vi "ManualControls_v4.vi"() -> ()   [LabVIEW 2013]
uses:
  <vilib>/Utility/miscctls.llb/LVPointTypeDef.ctl
  <vilib>/DAQmx/write.llb/DAQmx Write (Analog DBL 1Chan 1Samp).vi
  <vilib>/DAQmx/write.llb/DAQmx Write (Digital U32 1Chan 1Samp).vi
  <vilib>/DAQmx/miscellaneous.llb/DAQmx Fill In Error Info.vi
  DeviceVIs/Novatech/Novatech 409A.lvlib
panel:
  in  "Update Hardware":bool
  in  "?":enum32{"Controls", "File IO", "Errors"}(tab)
  in  "Master Output Bits":bool[](array[boolean])=[TRUE, TRUE, TRUE, TRUE, FALSE, FALSE, TRUE, FALSE, FALSE, FALSE, TRUE, FALSE, TRUE, TRUE, TRUE, TRUE, FALSE, FALSE, FALSE, FALSE, FALSE, FALSE, FALSE, FALSE]
  in  "Slave Output Bits":bool[](array[boolean])=[FALSE, FALSE, FALSE, FALSE, FALSE, FALSE, FALSE, FALSE, FALSE, FALSE, FALSE, FALSE, FALSE, FALSE, FALSE, FALSE, FALSE, FALSE, FALSE, FALSE, FALSE, FALSE, FALSE, FALSE]
  in  "Set Master":bool=TRUE
  in  "Set Slave":bool
  in  "AO Values":T1(array[cluster])=[{"DAQmx Global Channel"="AO0_0", "Numeric"=-9.792}, {"DAQmx Global Channel"="AO0_1", "Numeric"=-7.904}, {"DAQmx Global Channel"="AO0_2", "Numeric"=-3.981}, {"DAQmx Global Channel"="AO0_3", "Numeric"=-7.5}, {"DAQmx Global Channel"="AO0_4", "Numeric"=7.0}, {"DAQmx Global Channel"="AO0_5", "Numeric"=1.18}, {"DAQmx Global Channel"="AO0_6", "Numeric"=-8.918}, {"DAQmx Global Channel"="AO0_7", "Numeric"=1.1}, {"DAQmx Global Channel"="AO1_0", "Numeric"=8.0}, {"DAQmx Global Channel"="AO1_1", "Numeric"=0.45}, {"DAQmx Global Channel"="AO1_2", "Numeric"=1.3}, {"DAQmx Global Channel"="AO1_3", "Numeric"=0.0}, {"DAQmx Global Channel"="AO1_4", "Numeric"=0.3}, {"DAQmx Global Channel"="AO1_5", "Numeric"=1.2}, {"DAQmx Global Channel"="AO1_6", "Numeric"=1.6}, {"DAQmx Global Channel"="AO1_7", "Numeric"=0.12}, {"DAQmx Global Channel"="AO2_0", "Numeric"=0.0}, {"DAQmx Global Channel"="AO2_1", "Numeric"=0.0}, {"DAQmx Global Channel"="AO3_0", "Numeric"=0.0}, {"DAQmx Global Channel"="AO3_1", "Numeric"=0.0}, {"DAQmx Global Channel"="AO3_2", "Numeric"=0.0}, {"DAQmx Global Channel"="AO3_3", "Numeric"=0.0}, {"DAQmx Global Channel"="AO3_4", "Numeric"=0.0}, {"DAQmx Global Channel"="AO3_5", "Numeric"=0.0}, {"DAQmx Global Channel"="AO3_6", "Numeric"=0.0}, {"DAQmx Global Channel"="AO3_7", "Numeric"=0.0}] {"Numeric" step=1e-09 format="%_6g"}
  in  "Presets":T2(ring)
  in  "DO Values":T3(array[cluster])=[{"DAQmx Global Channel"="DO0_0", "DO Bits"=[TRUE, TRUE, FALSE, FALSE, FALSE, FALSE, TRUE, TRUE, FALSE, FALSE, FALSE, FALSE, FALSE, FALSE, FALSE, FALSE]}, {"DAQmx Global Channel"="DO1_0", "DO Bits"=[TRUE, FALSE, TRUE, TRUE, FALSE, TRUE, TRUE, TRUE, FALSE, FALSE, FALSE, FALSE, FALSE, FALSE, FALSE, FALSE]}, {"DAQmx Global Channel"="DO2_0", "DO Bits"=[]}, {"DAQmx Global Channel"="DO3_0", "DO Bits"=[]}]
  in  "Novatech settings":T4(array[cluster])
  in  "History":string(combo)
  in  "Save":bool
  in  "Load":bool
  in  "Path":path=path "C:/Experiment/Data Acquisition/Hardware Control/procedures/ManualControl"
  in  "error in":errorcluster
  out "error out":errorcluster
  # "Analog out"
  # "Digital Out"
  # "Ports are setup for 16 bit output, but only 16 are used"
  # "Master PB (PB 0)"
  # "Slave PB (PB 1)"
  # "Novatechs"
  # "0"
  # "8"
  # "12"
  # "4"
  # "16"
  # "20"
  # "0"
  # "8"
  # "12"
  # "4"
  # "16"
  # "20"
  # "Templates"
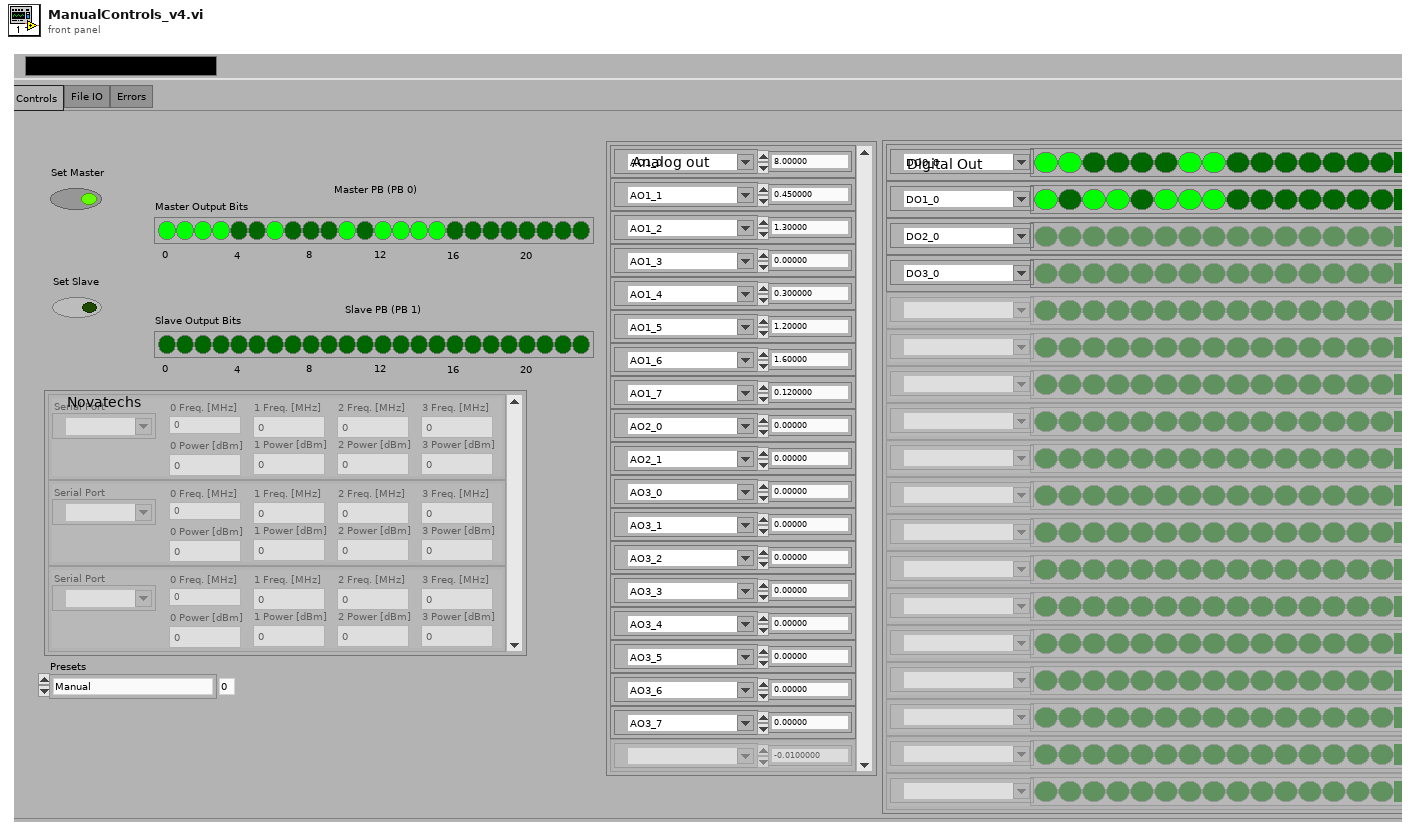
[diagram p1: front panel]
types:
  T1 = cluster{"DAQmx Global Channel":refnum<k21>, "Numeric":dbl}[]
  T2 = enum16{"Manual", "Rb MOT", "Yb MOT", "RbYb Warmup", "RbYb Turn Off", "Sr Warmup"}
  T3 = cluster{"DAQmx Global Channel":refnum<k21>, "DO Bits":bool[]}[]
  T4 = cluster{"0 Freq. [MHz]":dbl, "0 Power [dBm]":dbl, "Serial Port":refnum<visa-resource-name>, "1 Freq. [MHz]":dbl, "1 Power [dBm]":dbl, "2 Freq. [MHz]":dbl, "2 Power [dBm]":dbl, "3 Freq. [MHz]":dbl, "3 Power [dBm]":dbl}[]
  T5 = typedef "Semaphore RefNum" = refnum<k1>
  T6 = enum16{"open", "open or create", "create or replace", "create", "open (read only)"}
  T7 = enum16{"Always On", "Always Off", "Off While Running"}
  T8 = typedef "LVPointTypeDef.ctl" = cluster{"Horizontal":i16, "Vertical":i16}
  T9 = cluster{"Master Output Bits":bool[], "Slave Output Bits":bool[], "AO Values":cluster{"DAQmx Global Channel":refnum<k21>, "Numeric":dbl}[], "DO Values":cluster{"DAQmx Global Channel":refnum<k21>, "DO Bits":bool[]}[], "Novatech settings":cluster{"0 Freq. [MHz]":dbl, "0 Power [dBm]":dbl, "Serial Port":refnum<visa-resource-name>, "1 Freq. [MHz]":dbl, "1 Power [dBm]":dbl, "2 Freq. [MHz]":dbl, "2 Power [dBm]":dbl, "3 Freq. [MHz]":dbl, "3 Power [dBm]":dbl}[]}
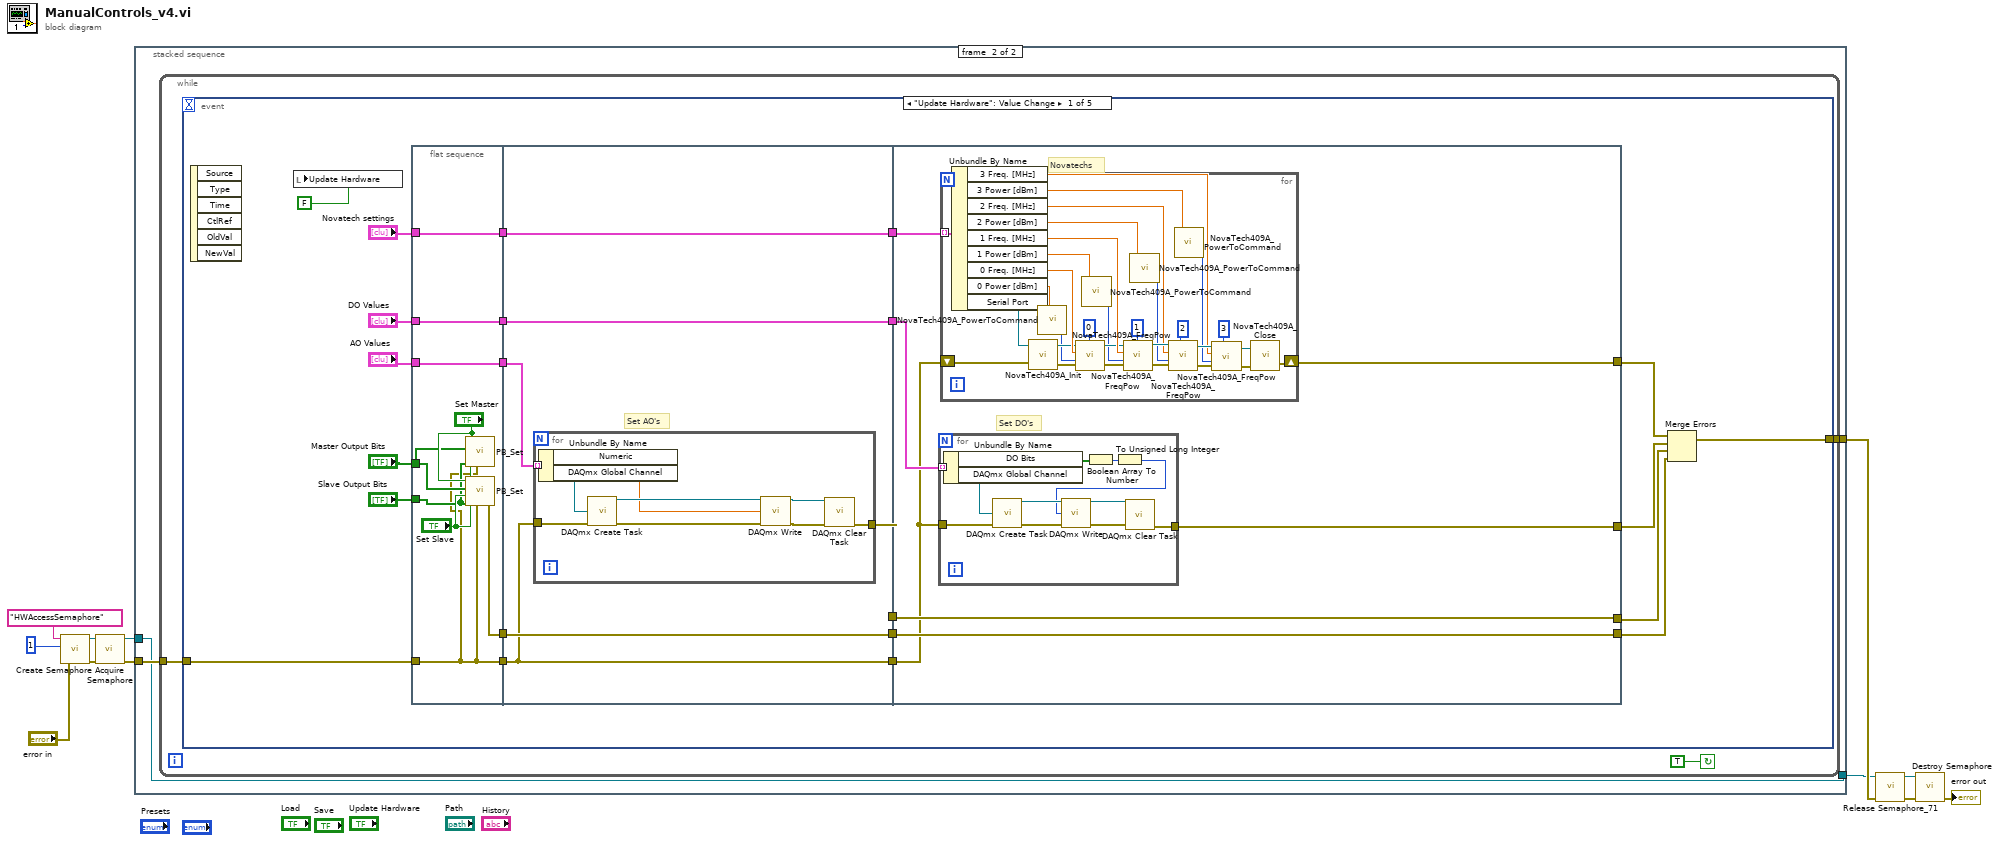
[diagram p0: block diagram]
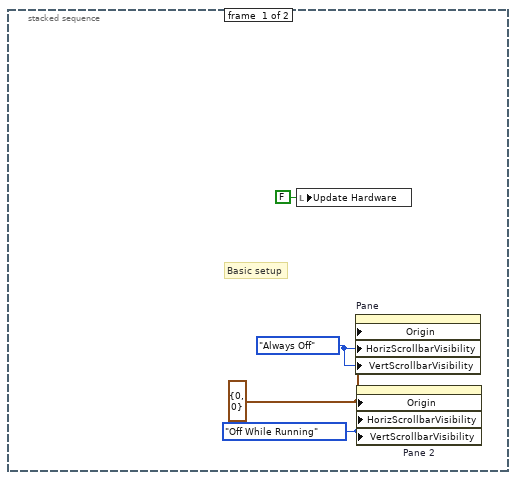
[diagram p2: hidden frame]
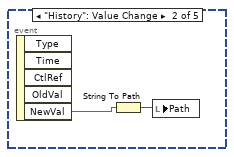
[diagram p3: hidden frame]
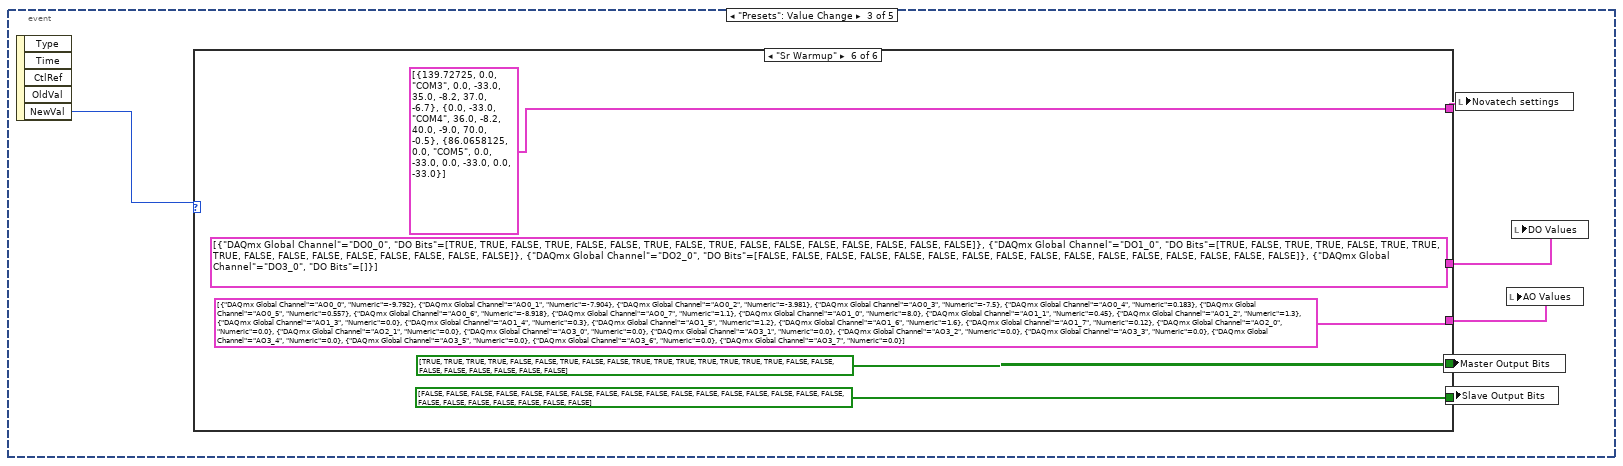
[diagram p4: hidden frame]
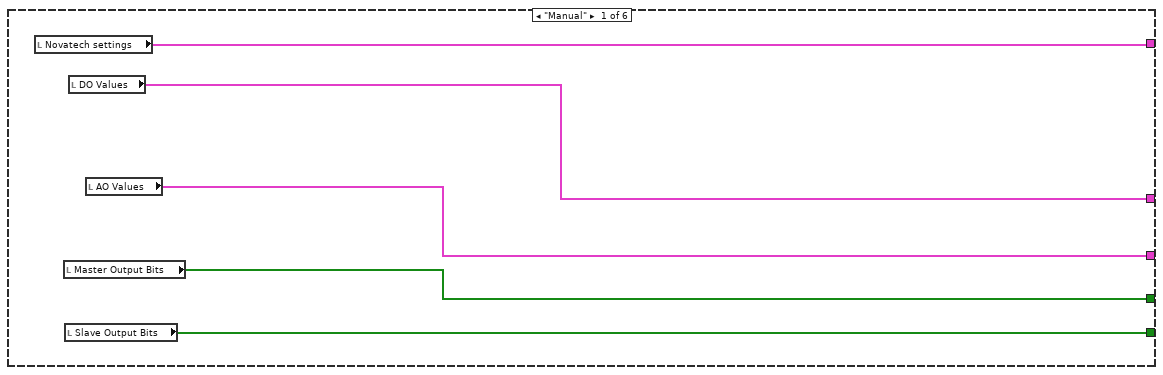
[diagram p5: hidden frame]
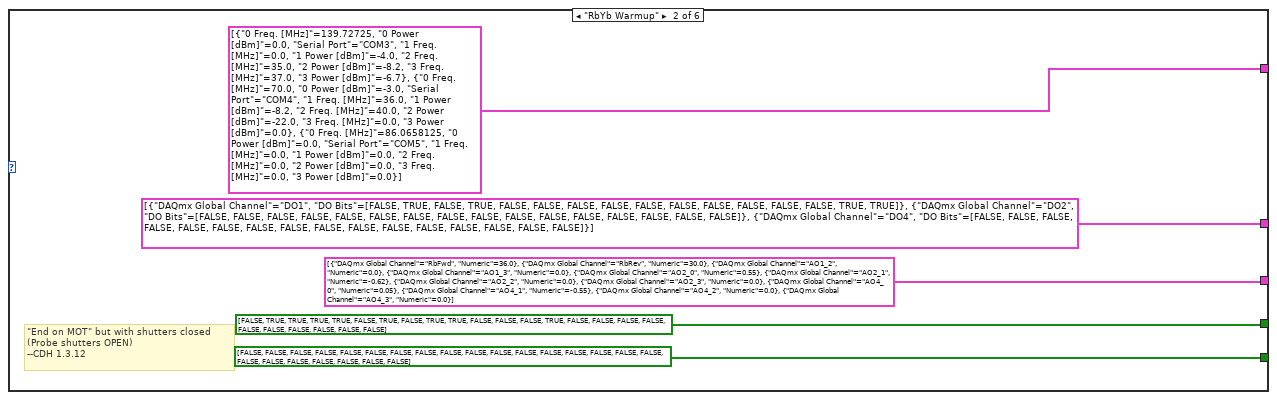
[diagram p6: hidden frame]
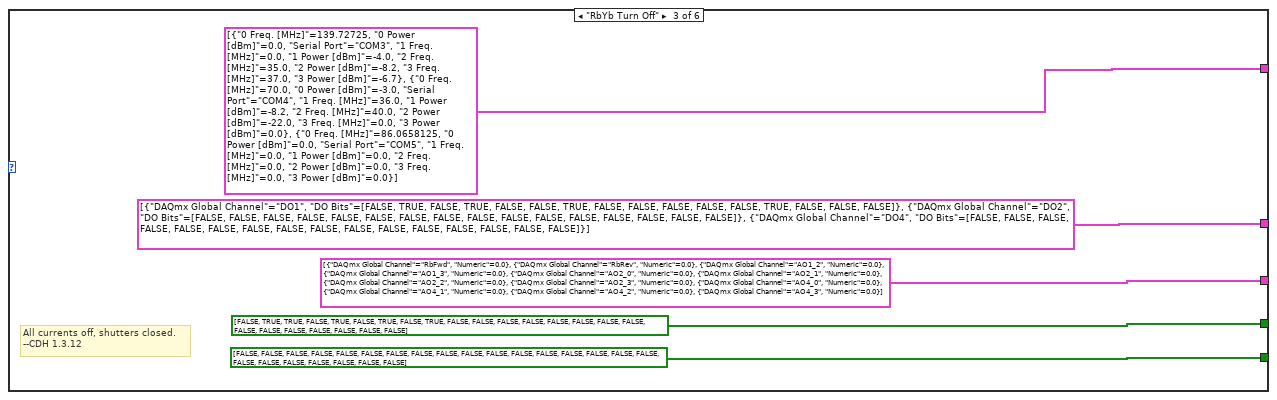
[diagram p7: hidden frame]
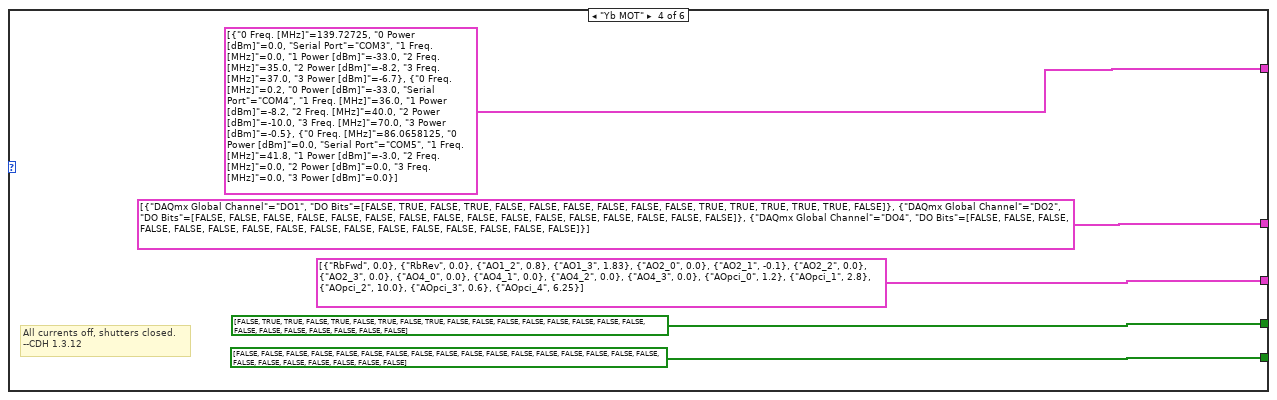
[diagram p8: hidden frame]
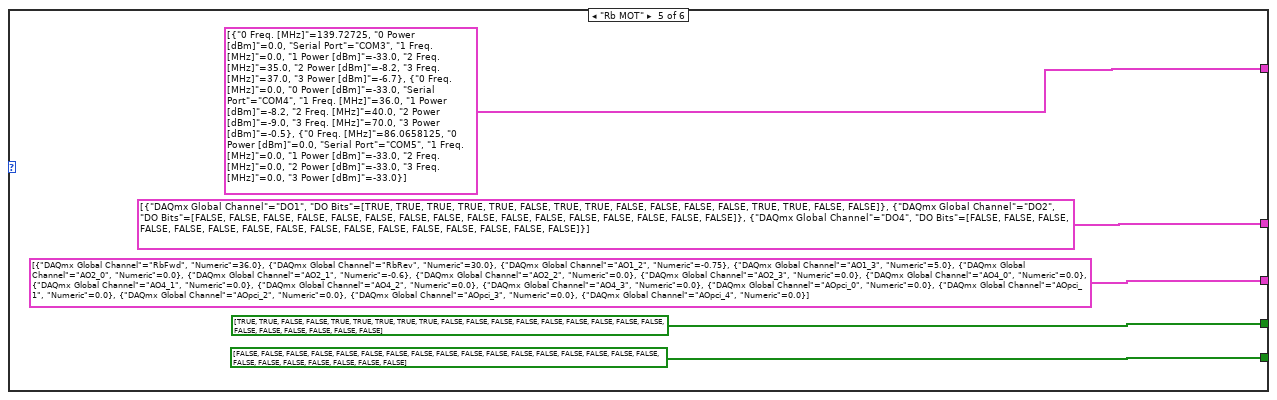
[diagram p9: hidden frame]
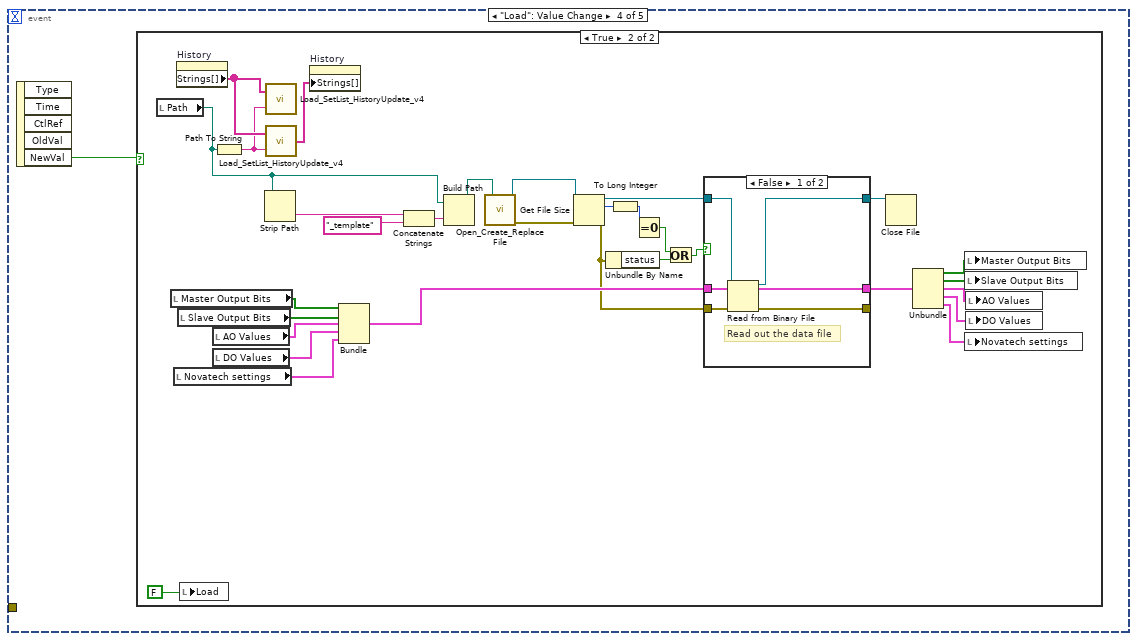
[diagram p10: hidden frame]
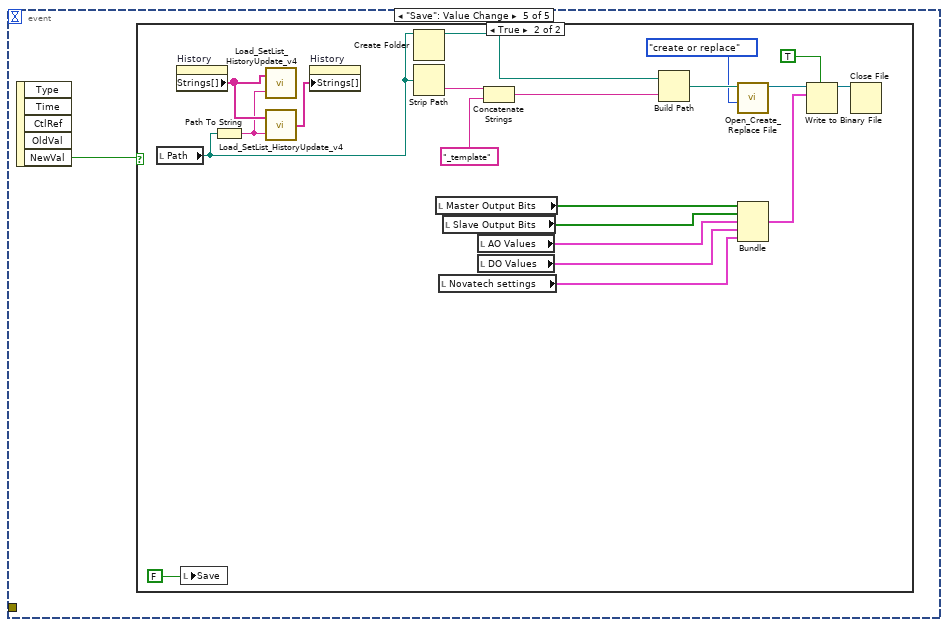
[diagram p13: hidden frame]
diagram:
  n1 = call <vilib>:"Create Semaphore.vi"("error in (no error)"="error in", "size (1)"=1, "name (unnamed)"="HWAccessSemaphore") -> ("error out"=w6:errorcluster, "semaphore"=w7:T5)  [unwired: 3 out]
  n2 = call <vilib>:"Acquire Semaphore.vi"("error in (no error)"=w6, "semaphore"=w7) -> ("error out"=w3:errorcluster, "semaphore out"=w2:T5)  [unwired: 1 in, 3 out]
  n3 = stacked-sequence {
    tunnel: [_ w19] -> w9
    tunnel: w3 -> [_ w18]
    tunnel: w2 -> [_ w17]
    tunnel: [_ w17] -> w1
    frame #0 {
      w16 = T7."Always Off" ("Horizontal Scrollbar Visibility")
      w15 = T8 {"Horizontal"=0, "Vertical"=0} ("Origin")
      w14 = T7."Off While Running" ("Horizontal Scrollbar Visibility")
      # "Basic setup"
      n4 = local write "Update Hardware"(FALSE ("Update Hardware")) -> ()
      n5 = property on="Pane" class="Pane"("Origin"=w15, "HorizScrollbarVisibility"=w16, "VertScrollbarVisibility"=w16) -> ()  [unwired: 2 in, 2 out]
      n6 = property on="Pane 2" class="Pane"("Origin"=w15, "HorizScrollbarVisibility"=w14, "VertScrollbarVisibility"=w14) -> ()  [unwired: 2 in, 2 out]
    }
    frame #1 {
      n7 = while {
        tunnel: [w22] -> w19
        tunnel: w18 -> [w21]
        stop <- TRUE continue-if-true
        n8 = event shown="[0] \"Update Hardware\": Value Change" {
          selector: _ -> [_ _ _ _ _]
          dyn-events: _ -> [_ _ _ _ _]
          timeout: _ -> [_ _ _ _ _]
          tunnel: [w44 _ _ _ _] -> w22
          tunnel: w21 -> [w43 _ _ _ _]
          event "Update Hardware": Value Change {
            n9 = event-data() -> ()  [unwired: 1 in, 6 out]
            n10 = local write "Update Hardware"(FALSE) -> ()
            n11 = flat-sequence {
              tunnel: [w45] -> w42
              tunnel: [w51] -> w41
              tunnel: "AO Values" -> [w51]
              tunnel: "Master Output Bits" -> [w50]
              tunnel: "Slave Output Bits" -> [w49]
              tunnel: "DO Values" -> [w47]
              tunnel: "Novatech settings" -> [w48]
              tunnel: [w47] -> w40
              tunnel: [w48] -> w39
              tunnel: w43 -> [w46]
              tunnel: [w46] -> w38
              tunnel: w42 -> [w55]
              tunnel: w41 -> [w58]
              tunnel: [w59] -> w37
              tunnel: w40 -> [w57]
              tunnel: [w57] -> w36
              tunnel: [w56] -> w35
              tunnel: w39 -> [w56]
              tunnel: [w54] -> w34
              tunnel: w38 -> [w54]
              tunnel: [w55] -> w33
              tunnel: [w75] -> w31
              tunnel: w37 -> [w70]
              tunnel: w36 -> [w74]
              tunnel: [w73] -> w32
              tunnel: w35 -> [w72]
              tunnel: w34 -> [w69]
              tunnel: [w71] -> w24
              tunnel: w33 -> [w71]
              tunnel: [w70] -> w25
              frame #0 {
                # "Set PulseBlaster"
                n12 = call "PB_Set.vi"("Set Master"="Set Master", "Master Output Bits"=w50, "Set Slave"="Set Slave", "Slave Output Bits"=w49, "error in"=w46) -> ()  [unwired: 3 out]
                n13 = call "PB_Set.vi"("Set Master"="Set Master", "Master Output Bits"=w50, "Set Slave"="Set Slave", "Slave Output Bits"=w49, "error in"=w46) -> ("error out"=w45:errorcluster)  [unwired: 2 out]
              }
              frame #1 {
                # "Set AO's"
                n14 = for {
                  tunnel: [w66] -> w59
                  tunnel: w54 -> [w65]
                  tunnel: w58 -> [w62] mode=indexing
                  n15 = Unbundle By Name(w62) -> ("Numeric"=w61:dbl, "DAQmx Global Channel"=w60:refnum<k21>)
                  n16 = call <vilib>:"DAQmx Create Task.vi"("global virtual channels"=w60, "error in"=w65) -> ("task out"=w63:refnum<k21>, "error out"=w64:errorcluster)  [unwired: 3 in, 9 out]
                  n17 = call-poly <vilib>:"DAQmx Write.vi"("task/channels in"=w63, "data"=w61, "error in"=w64) -> ("task out"=w68:refnum<k21>, "error out"=w67:errorcluster)  [unwired: 1 in, 10 out]
                  n18 = call <vilib>:"DAQmx Clear Task.vi"("task in"=w68, "error in"=w67) -> ("error out"=w66:errorcluster)  [unwired: 13 out]
                }
              }
              frame #2 {
                # "Novatechs"
                # "Set DO's"
                n19 = for {
                  tunnel: [w114] -> w75
                  tunnel: w69 -> [w113]
                  tunnel: w74 -> [w110] mode=indexing
                  n20 = Unbundle By Name(w110) -> ("DO Bits"=w107:bool[], "DAQmx Global Channel"=w109:refnum<k21>)
                  n21 = call <vilib>:"DAQmx Create Task.vi"("global virtual channels"=w109, "error in"=w113) -> ("task out"=w111:refnum<k21>, "error out"=w112:errorcluster)  [unwired: 3 in, 9 out]
                  n22 = Boolean Array To Number(Boolean array=w107) -> (number=w108:u32)
                  n23 = To Unsigned Long Integer(number=w108) -> (unsigned 32bit integer=w106:u32)
                  n24 = call-poly <vilib>:"DAQmx Write.vi"("task/channels in"=w111, "data"=w106, "error in"=w112) -> ("task out"=w116:refnum<k21>, "error out"=w115:errorcluster)  [unwired: 1 in, 10 out]
                  n25 = call <vilib>:"DAQmx Clear Task.vi"("task in"=w116, "error in"=w115) -> ("error out"=w114:errorcluster)  [unwired: 13 out]
                }
                n26 = for {
                  tunnel: w72 -> [w105] mode=indexing
                  shift-right: [w91] -> w73
                  shift-left: w69 -> [w103]
                  n27 = Unbundle By Name(w105) -> ("3 Freq. [MHz]"=w84:dbl, "3 Power [dBm]"=w83:dbl, "2 Freq. [MHz]"=w85:dbl, "2 Power [dBm]"=w80:dbl, "1 Freq. [MHz]"=w98:dbl, "1 Power [dBm]"=w78:dbl, "0 Freq. [MHz]"=w100:dbl, "0 Power [dBm]"=w76:dbl, "Serial Port"=w104:refnum<visa-resource-name>)
                  n28 = call "NovaTech409A_Init.vi"("error in (no error)"=w103, "VISA resource name"=w104) -> ("error out"=w102:errorcluster, "VISA resource name out"=w99:refnum<visa-resource-name>)  [unwired: 1 in]
                  n29 = call "NovaTech409A_PowerToCommand.vi"("Novatech Power [dBm]"=w76) -> ("Novatech Command"=w77:u16)
                  n30 = call "NovaTech409A_FreqPow.vi"("VISA resource name"=w99, "Freq"=w100, "Power"=w77, "error in (no error)"=w102, "Channel (0-3)"=u8 0) -> ("VISA resource name out"=w97:refnum<visa-resource-name>, "error out"=w101:errorcluster)
                  n31 = call "NovaTech409A_PowerToCommand.vi"("Novatech Power [dBm]"=w78) -> ("Novatech Command"=w79:u16)
                  n32 = call "NovaTech409A_FreqPow.vi"("VISA resource name"=w97, "Freq"=w98, "Power"=w79, "error in (no error)"=w101, "Channel (0-3)"=u8 1) -> ("VISA resource name out"=w90:refnum<visa-resource-name>, "error out"=w94:errorcluster)
                  n33 = call "NovaTech409A_PowerToCommand.vi"("Novatech Power [dBm]"=w80) -> ("Novatech Command"=w81:u16)
                  n34 = call "NovaTech409A_FreqPow.vi"("VISA resource name"=w90, "Freq"=w85, "Power"=w81, "error in (no error)"=w94, "Channel (0-3)"=u8 2) -> ("VISA resource name out"=w89:refnum<visa-resource-name>, "error out"=w93:errorcluster)
                  n35 = call "NovaTech409A_PowerToCommand.vi"("Novatech Power [dBm]"=w83) -> ("Novatech Command"=w82:u16)
                  n36 = call "NovaTech409A_FreqPow.vi"("VISA resource name"=w89, "Freq"=w84, "Power"=w82, "error in (no error)"=w93, "Channel (0-3)"=u8 3) -> ("VISA resource name out"=w88:refnum<visa-resource-name>, "error out"=w92:errorcluster)
                  n37 = call "NovaTech409A_Close.vi"("error in (no error)"=w92, "VISA resource name"=w88) -> ("error out"=w91:errorcluster)  [unwired: 1 out]
                }
              }
            }
            n38 = Merge Errors(w32, w31, w25, w24) -> (w44:errorcluster)
          }
          event "History": Value Change {
            n39 = event-data() -> ("NewVal"=w118:string)  [unwired: 1 in, 4 out]
            n40 = String To Path(string=w118) -> (path=w117:path)
            n41 = local write "Path"(w117) -> ()
          }
          event "Presets": Value Change {
            n42 = event-data() -> ("NewVal"=w119:T2)  [unwired: 1 in, 4 out]
            n43 = case shown="\"Sr Warmup\"" w119 {
              tunnel: [w127 T1 [{"DAQmx Global Channel"="RbFwd", "Numeric"=36.0}, {"DAQmx Global Channel"="RbRev", "Numeric"=30.0}, {"DAQmx Global Channel"="AO1_2", "Numeric"=0.0}, {"DAQmx Global Channel"="AO1_3", "Numeric"=0.0}, {"DAQmx Global Channel"="AO2_0", "Numeric"=0.55}, {"DAQmx Global Channel"="AO2_1", "Numeric"=-0.62}, {"DAQmx Global Channel"="AO2_2", "Numeric"=0.0}, {"DAQmx Global Channel"="AO2_3", "Numeric"=0.0}, {"DAQmx Global Channel"="AO4_0", "Numeric"=0.05}, {"DAQmx Global Channel"="AO4_1", "Numeric"=-0.55}, {"DAQmx Global Channel"="AO4_2", "Numeric"=0.0}, {"DAQmx Global Channel"="AO4_3", "Numeric"=0.0}] ("AO Values") T1 [{"DAQmx Global Channel"="RbFwd", "Numeric"=0.0}, {"DAQmx Global Channel"="RbRev", "Numeric"=0.0}, {"DAQmx Global Channel"="AO1_2", "Numeric"=0.0}, {"DAQmx Global Channel"="AO1_3", "Numeric"=0.0}, {"DAQmx Global Channel"="AO2_0", "Numeric"=0.0}, {"DAQmx Global Channel"="AO2_1", "Numeric"=0.0}, {"DAQmx Global Channel"="AO2_2", "Numeric"=0.0}, {"DAQmx Global Channel"="AO2_3", "Numeric"=0.0}, {"DAQmx Global Channel"="AO4_0", "Numeric"=0.0}, {"DAQmx Global Channel"="AO4_1", "Numeric"=0.0}, {"DAQmx Global Channel"="AO4_2", "Numeric"=0.0}, {"DAQmx Global Channel"="AO4_3", "Numeric"=0.0}] ("AO Values") T1 [{"DAQmx Global Channel"="RbFwd", "Numeric"=0.0}, {"DAQmx Global Channel"="RbRev", "Numeric"=0.0}, {"DAQmx Global Channel"="AO1_2", "Numeric"=0.8}, {"DAQmx Global Channel"="AO1_3", "Numeric"=1.83}, {"DAQmx Global Channel"="AO2_0", "Numeric"=0.0}, {"DAQmx Global Channel"="AO2_1", "Numeric"=-0.1}, {"DAQmx Global Channel"="AO2_2", "Numeric"=0.0}, {"DAQmx Global Channel"="AO2_3", "Numeric"=0.0}, {"DAQmx Global Channel"="AO4_0", "Numeric"=0.0}, {"DAQmx Global Channel"="AO4_1", "Numeric"=0.0}, {"DAQmx Global Channel"="AO4_2", "Numeric"=0.0}, {"DAQmx Global Channel"="AO4_3", "Numeric"=0.0}, {"DAQmx Global Channel"="AOpci_0", "Numeric"=1.2}, {"DAQmx Global Channel"="AOpci_1", "Numeric"=2.8}, {"DAQmx Global Channel"="AOpci_2", "Numeric"=10.0}, {"DAQmx Global Channel"="AOpci_3", "Numeric"=0.6}, {"DAQmx Global Channel"="AOpci_4", "Numeric"=6.25}] ("AO Values") T1 [{"DAQmx Global Channel"="RbFwd", "Numeric"=36.0}, {"DAQmx Global Channel"="RbRev", "Numeric"=30.0}, {"DAQmx Global Channel"="AO1_2", "Numeric"=-0.75}, {"DAQmx Global Channel"="AO1_3", "Numeric"=5.0}, {"DAQmx Global Channel"="AO2_0", "Numeric"=0.0}, {"DAQmx Global Channel"="AO2_1", "Numeric"=-0.6}, {"DAQmx Global Channel"="AO2_2", "Numeric"=0.0}, {"DAQmx Global Channel"="AO2_3", "Numeric"=0.0}, {"DAQmx Global Channel"="AO4_0", "Numeric"=0.0}, {"DAQmx Global Channel"="AO4_1", "Numeric"=0.0}, {"DAQmx Global Channel"="AO4_2", "Numeric"=0.0}, {"DAQmx Global Channel"="AO4_3", "Numeric"=0.0}, {"DAQmx Global Channel"="AOpci_0", "Numeric"=0.0}, {"DAQmx Global Channel"="AOpci_1", "Numeric"=0.0}, {"DAQmx Global Channel"="AOpci_2", "Numeric"=0.0}, {"DAQmx Global Channel"="AOpci_3", "Numeric"=0.0}, {"DAQmx Global Channel"="AOpci_4", "Numeric"=0.0}] ("AO Values") T1 [{"DAQmx Global Channel"="AO0_0", "Numeric"=-9.792}, {"DAQmx Global Channel"="AO0_1", "Numeric"=-7.904}, {"DAQmx Global Channel"="AO0_2", "Numeric"=-3.981}, {"DAQmx Global Channel"="AO0_3", "Numeric"=-7.5}, {"DAQmx Global Channel"="AO0_4", "Numeric"=0.183}, {"DAQmx Global Channel"="AO0_5", "Numeric"=0.557}, {"DAQmx Global Channel"="AO0_6", "Numeric"=-8.918}, {"DAQmx Global Channel"="AO0_7", "Numeric"=1.1}, {"DAQmx Global Channel"="AO1_0", "Numeric"=8.0}, {"DAQmx Global Channel"="AO1_1", "Numeric"=0.45}, {"DAQmx Global Channel"="AO1_2", "Numeric"=1.3}, {"DAQmx Global Channel"="AO1_3", "Numeric"=0.0}, {"DAQmx Global Channel"="AO1_4", "Numeric"=0.3}, {"DAQmx Global Channel"="AO1_5", "Numeric"=1.2}, {"DAQmx Global Channel"="AO1_6", "Numeric"=1.6}, {"DAQmx Global Channel"="AO1_7", "Numeric"=0.12}, {"DAQmx Global Channel"="AO2_0", "Numeric"=0.0}, {"DAQmx Global Channel"="AO2_1", "Numeric"=0.0}, {"DAQmx Global Channel"="AO3_0", "Numeric"=0.0}, {"DAQmx Global Channel"="AO3_1", "Numeric"=0.0}, {"DAQmx Global Channel"="AO3_2", "Numeric"=0.0}, {"DAQmx Global Channel"="AO3_3", "Numeric"=0.0}, {"DAQmx Global Channel"="AO3_4", "Numeric"=0.0}, {"DAQmx Global Channel"="AO3_5", "Numeric"=0.0}, {"DAQmx Global Channel"="AO3_6", "Numeric"=0.0}, {"DAQmx Global Channel"="AO3_7", "Numeric"=0.0}] ("AO Values")] -> w122
              tunnel: [w126 bool[] [FALSE, TRUE, TRUE, TRUE, TRUE, FALSE, TRUE, FALSE, TRUE, TRUE, FALSE, FALSE, FALSE, TRUE, FALSE, FALSE, FALSE, FALSE, FALSE, FALSE, FALSE, FALSE, FALSE, FALSE] ("Master Output Bits") bool[] [FALSE, TRUE, TRUE, FALSE, TRUE, FALSE, TRUE, FALSE, TRUE, FALSE, FALSE, FALSE, FALSE, FALSE, FALSE, FALSE, FALSE, FALSE, FALSE, FALSE, FALSE, FALSE, FALSE, FALSE] ("Master Output Bits") bool[] [FALSE, TRUE, TRUE, FALSE, TRUE, FALSE, TRUE, FALSE, TRUE, FALSE, FALSE, FALSE, FALSE, FALSE, FALSE, FALSE, FALSE, FALSE, FALSE, FALSE, FALSE, FALSE, FALSE, FALSE] ("Master Output Bits") bool[] [TRUE, TRUE, FALSE, FALSE, TRUE, TRUE, TRUE, TRUE, TRUE, FALSE, FALSE, FALSE, FALSE, FALSE, FALSE, FALSE, FALSE, FALSE, FALSE, FALSE, FALSE, FALSE, FALSE, FALSE] ("Master Output Bits") bool[] [TRUE, TRUE, TRUE, TRUE, FALSE, FALSE, TRUE, FALSE, FALSE, TRUE, TRUE, TRUE, TRUE, TRUE, TRUE, TRUE, FALSE, FALSE, FALSE, FALSE, FALSE, FALSE, FALSE, FALSE] ("Master Output Bits")] -> w120
              tunnel: [w125 bool[] [FALSE, FALSE, FALSE, FALSE, FALSE, FALSE, FALSE, FALSE, FALSE, FALSE, FALSE, FALSE, FALSE, FALSE, FALSE, FALSE, FALSE, FALSE, FALSE, FALSE, FALSE, FALSE, FALSE, FALSE] ("Slave Output Bits") bool[] [FALSE, FALSE, FALSE, FALSE, FALSE, FALSE, FALSE, FALSE, FALSE, FALSE, FALSE, FALSE, FALSE, FALSE, FALSE, FALSE, FALSE, FALSE, FALSE, FALSE, FALSE, FALSE, FALSE, FALSE] ("Slave Output Bits") bool[] [FALSE, FALSE, FALSE, FALSE, FALSE, FALSE, FALSE, FALSE, FALSE, FALSE, FALSE, FALSE, FALSE, FALSE, FALSE, FALSE, FALSE, FALSE, FALSE, FALSE, FALSE, FALSE, FALSE, FALSE] ("Slave Output Bits") bool[] [FALSE, FALSE, FALSE, FALSE, FALSE, FALSE, FALSE, FALSE, FALSE, FALSE, FALSE, FALSE, FALSE, FALSE, FALSE, FALSE, FALSE, FALSE, FALSE, FALSE, FALSE, FALSE, FALSE, FALSE] ("Slave Output Bits") bool[] [FALSE, FALSE, FALSE, FALSE, FALSE, FALSE, FALSE, FALSE, FALSE, FALSE, FALSE, FALSE, FALSE, FALSE, FALSE, FALSE, FALSE, FALSE, FALSE, FALSE, FALSE, FALSE, FALSE, FALSE] ("Slave Output Bits")] -> w121
              tunnel: [w128 T3 [{"DAQmx Global Channel"="DO1", "DO Bits"=[FALSE, TRUE, FALSE, TRUE, FALSE, FALSE, FALSE, FALSE, FALSE, FALSE, FALSE, FALSE, FALSE, FALSE, TRUE, TRUE]}, {"DAQmx Global Channel"="DO2", "DO Bits"=[FALSE, FALSE, FALSE, FALSE, FALSE, FALSE, FALSE, FALSE, FALSE, FALSE, FALSE, FALSE, FALSE, FALSE, FALSE, FALSE]}, {"DAQmx Global Channel"="DO4", "DO Bits"=[FALSE, FALSE, FALSE, FALSE, FALSE, FALSE, FALSE, FALSE, FALSE, FALSE, FALSE, FALSE, FALSE, FALSE, FALSE, FALSE]}] ("DO Values") T3 [{"DAQmx Global Channel"="DO1", "DO Bits"=[FALSE, TRUE, FALSE, TRUE, FALSE, FALSE, TRUE, FALSE, FALSE, FALSE, FALSE, FALSE, TRUE, FALSE, FALSE, FALSE]}, {"DAQmx Global Channel"="DO2", "DO Bits"=[FALSE, FALSE, FALSE, FALSE, FALSE, FALSE, FALSE, FALSE, FALSE, FALSE, FALSE, FALSE, FALSE, FALSE, FALSE, FALSE]}, {"DAQmx Global Channel"="DO4", "DO Bits"=[FALSE, FALSE, FALSE, FALSE, FALSE, FALSE, FALSE, FALSE, FALSE, FALSE, FALSE, FALSE, FALSE, FALSE, FALSE, FALSE]}] ("DO Values") T3 [{"DAQmx Global Channel"="DO1", "DO Bits"=[FALSE, TRUE, FALSE, TRUE, FALSE, FALSE, FALSE, FALSE, FALSE, FALSE, TRUE, TRUE, TRUE, TRUE, TRUE, FALSE]}, {"DAQmx Global Channel"="DO2", "DO Bits"=[FALSE, FALSE, FALSE, FALSE, FALSE, FALSE, FALSE, FALSE, FALSE, FALSE, FALSE, FALSE, FALSE, FALSE, FALSE, FALSE]}, {"DAQmx Global Channel"="DO4", "DO Bits"=[FALSE, FALSE, FALSE, FALSE, FALSE, FALSE, FALSE, FALSE, FALSE, FALSE, FALSE, FALSE, FALSE, FALSE, FALSE, FALSE]}] ("DO Values") T3 [{"DAQmx Global Channel"="DO1", "DO Bits"=[TRUE, TRUE, TRUE, TRUE, TRUE, FALSE, TRUE, TRUE, FALSE, FALSE, FALSE, FALSE, TRUE, TRUE, FALSE, FALSE]}, {"DAQmx Global Channel"="DO2", "DO Bits"=[FALSE, FALSE, FALSE, FALSE, FALSE, FALSE, FALSE, FALSE, FALSE, FALSE, FALSE, FALSE, FALSE, FALSE, FALSE, FALSE]}, {"DAQmx Global Channel"="DO4", "DO Bits"=[FALSE, FALSE, FALSE, FALSE, FALSE, FALSE, FALSE, FALSE, FALSE, FALSE, FALSE, FALSE, FALSE, FALSE, FALSE, FALSE]}] ("DO Values") T3 [{"DAQmx Global Channel"="DO0_0", "DO Bits"=[TRUE, TRUE, FALSE, TRUE, FALSE, FALSE, TRUE, FALSE, TRUE, FALSE, FALSE, FALSE, FALSE, FALSE, FALSE, FALSE]}, {"DAQmx Global Channel"="DO1_0", "DO Bits"=[TRUE, FALSE, TRUE, TRUE, FALSE, TRUE, TRUE, TRUE, FALSE, FALSE, FALSE, FALSE, FALSE, FALSE, FALSE, FALSE]}, {"DAQmx Global Channel"="DO2_0", "DO Bits"=[FALSE, FALSE, FALSE, FALSE, FALSE, FALSE, FALSE, FALSE, FALSE, FALSE, FALSE, FALSE, FALSE, FALSE, FALSE, FALSE]}, {"DAQmx Global Channel"="DO3_0", "DO Bits"=[]}] ("DO Values")] -> w123
              tunnel: [w129 T4 [{"0 Freq. [MHz]"=139.72725, "0 Power [dBm]"=0.0, "Serial Port"="COM3", "1 Freq. [MHz]"=0.0, "1 Power [dBm]"=-4.0, "2 Freq. [MHz]"=35.0, "2 Power [dBm]"=-8.2, "3 Freq. [MHz]"=37.0, "3 Power [dBm]"=-6.7}, {"0 Freq. [MHz]"=70.0, "0 Power [dBm]"=-3.0, "Serial Port"="COM4", "1 Freq. [MHz]"=36.0, "1 Power [dBm]"=-8.2, "2 Freq. [MHz]"=40.0, "2 Power [dBm]"=-22.0, "3 Freq. [MHz]"=0.0, "3 Power [dBm]"=0.0}, {"0 Freq. [MHz]"=86.0658125, "0 Power [dBm]"=0.0, "Serial Port"="COM5", "1 Freq. [MHz]"=0.0, "1 Power [dBm]"=0.0, "2 Freq. [MHz]"=0.0, "2 Power [dBm]"=0.0, "3 Freq. [MHz]"=0.0, "3 Power [dBm]"=0.0}] ("Novatech settings") T4 [{"0 Freq. [MHz]"=139.72725, "0 Power [dBm]"=0.0, "Serial Port"="COM3", "1 Freq. [MHz]"=0.0, "1 Power [dBm]"=-4.0, "2 Freq. [MHz]"=35.0, "2 Power [dBm]"=-8.2, "3 Freq. [MHz]"=37.0, "3 Power [dBm]"=-6.7}, {"0 Freq. [MHz]"=70.0, "0 Power [dBm]"=-3.0, "Serial Port"="COM4", "1 Freq. [MHz]"=36.0, "1 Power [dBm]"=-8.2, "2 Freq. [MHz]"=40.0, "2 Power [dBm]"=-22.0, "3 Freq. [MHz]"=0.0, "3 Power [dBm]"=0.0}, {"0 Freq. [MHz]"=86.0658125, "0 Power [dBm]"=0.0, "Serial Port"="COM5", "1 Freq. [MHz]"=0.0, "1 Power [dBm]"=0.0, "2 Freq. [MHz]"=0.0, "2 Power [dBm]"=0.0, "3 Freq. [MHz]"=0.0, "3 Power [dBm]"=0.0}] ("Novatech settings") T4 [{"0 Freq. [MHz]"=139.72725, "0 Power [dBm]"=0.0, "Serial Port"="COM3", "1 Freq. [MHz]"=0.0, "1 Power [dBm]"=-33.0, "2 Freq. [MHz]"=35.0, "2 Power [dBm]"=-8.2, "3 Freq. [MHz]"=37.0, "3 Power [dBm]"=-6.7}, {"0 Freq. [MHz]"=0.2, "0 Power [dBm]"=-33.0, "Serial Port"="COM4", "1 Freq. [MHz]"=36.0, "1 Power [dBm]"=-8.2, "2 Freq. [MHz]"=40.0, "2 Power [dBm]"=-10.0, "3 Freq. [MHz]"=70.0, "3 Power [dBm]"=-0.5}, {"0 Freq. [MHz]"=86.0658125, "0 Power [dBm]"=0.0, "Serial Port"="COM5", "1 Freq. [MHz]"=41.8, "1 Power [dBm]"=-3.0, "2 Freq. [MHz]"=0.0, "2 Power [dBm]"=0.0, "3 Freq. [MHz]"=0.0, "3 Power [dBm]"=0.0}] ("Novatech settings") T4 [{"0 Freq. [MHz]"=139.72725, "0 Power [dBm]"=0.0, "Serial Port"="COM3", "1 Freq. [MHz]"=0.0, "1 Power [dBm]"=-33.0, "2 Freq. [MHz]"=35.0, "2 Power [dBm]"=-8.2, "3 Freq. [MHz]"=37.0, "3 Power [dBm]"=-6.7}, {"0 Freq. [MHz]"=0.0, "0 Power [dBm]"=-33.0, "Serial Port"="COM4", "1 Freq. [MHz]"=36.0, "1 Power [dBm]"=-8.2, "2 Freq. [MHz]"=40.0, "2 Power [dBm]"=-9.0, "3 Freq. [MHz]"=70.0, "3 Power [dBm]"=-0.5}, {"0 Freq. [MHz]"=86.0658125, "0 Power [dBm]"=0.0, "Serial Port"="COM5", "1 Freq. [MHz]"=0.0, "1 Power [dBm]"=-33.0, "2 Freq. [MHz]"=0.0, "2 Power [dBm]"=-33.0, "3 Freq. [MHz]"=0.0, "3 Power [dBm]"=-33.0}] ("Novatech settings") T4 [{"0 Freq. [MHz]"=139.72725, "0 Power [dBm]"=0.0, "Serial Port"="COM3", "1 Freq. [MHz]"=0.0, "1 Power [dBm]"=-33.0, "2 Freq. [MHz]"=35.0, "2 Power [dBm]"=-8.2, "3 Freq. [MHz]"=37.0, "3 Power [dBm]"=-6.7}, {"0 Freq. [MHz]"=0.0, "0 Power [dBm]"=-33.0, "Serial Port"="COM4", "1 Freq. [MHz]"=36.0, "1 Power [dBm]"=-8.2, "2 Freq. [MHz]"=40.0, "2 Power [dBm]"=-9.0, "3 Freq. [MHz]"=70.0, "3 Power [dBm]"=-0.5}, {"0 Freq. [MHz]"=86.0658125, "0 Power [dBm]"=0.0, "Serial Port"="COM5", "1 Freq. [MHz]"=0.0, "1 Power [dBm]"=-33.0, "2 Freq. [MHz]"=0.0, "2 Power [dBm]"=-33.0, "3 Freq. [MHz]"=0.0, "3 Power [dBm]"=-33.0}] ("Novatech settings")] -> w124
              frame "Manual" {
                n44 = local read "Novatech settings"() -> (w129:T4)
                n45 = local read "Master Output Bits"() -> (w126:bool[])
                n46 = local read "Slave Output Bits"() -> (w125:bool[])
                n47 = local read "DO Values"() -> (w128:T3)
                n48 = local read "AO Values"() -> (w127:T1)
              }
              frame "RbYb Warmup" {
                # "\"End on MOT\" but with shutters closed\n(Probe shutters OPEN)\n--CDH 1.3.12"
              }
              frame "RbYb Turn Off" {
                # "All currents off, shutters closed.\n--CDH 1.3.12"
              }
              frame "Yb MOT" {
                # "All currents off, shutters closed.\n--CDH 1.3.12"
              }
              frame "Rb MOT" {
              }
              frame "Sr Warmup" {
              }
            }
            n49 = local write "Master Output Bits"(w120) -> ()
            n50 = local write "Slave Output Bits"(w121) -> ()
            n51 = local write "Novatech settings"(w124) -> ()
            n52 = local write "AO Values"(w122) -> ()
            n53 = local write "DO Values"(w123) -> ()
          }
          event "Load": Value Change {
            n54 = event-data() -> ("NewVal"=w155:bool)  [unwired: 1 in, 4 out]
            n55 = case shown="True" w155 {
              frame False {
              }
              frame True {
                n56 = local read "Path"() -> (w160:path)
                n57 = local read "Master Output Bits"() -> (w183:bool[])
                n58 = local read "Novatech settings"() -> (w179:T4)
                n59 = property on="History" class="CmbBox"() -> ("Strings[]"=w186:string[])  [unwired: 2 in, 2 out]
                n60 = local read "Slave Output Bits"() -> (w182:bool[])
                n61 = local write "Load"(FALSE) -> ()
                n62 = local read "AO Values"() -> (w181:T1)
                n63 = local read "DO Values"() -> (w180:T3)
                n64 = Path To String(path=w160) -> (string=w185:string)
                n65 = Strip Path(path=w160) -> (name=w161:string)  [unwired: 1 out]
                n66 = call "Load_SetList_HistoryUpdate_v4.vi"("New Element"=w185, "History in"=w186) -> ()  [unwired: 1 out]
                n67 = call "Load_SetList_HistoryUpdate_v4.vi"("New Element"=w185, "History in"=w186) -> ("History Out"=w156:string[])
                n68 = property on="History" class="CmbBox"("Strings[]"=w156) -> ()  [unwired: 2 in, 2 out]
                n69 = Bundle("Master Output Bits"=w183, "Slave Output Bits"=w182, "AO Values"=w181, "DO Values"=w180, "Novatech settings"=w179) -> (w162:T9)  [unwired: 1 in]
                n70 = Concatenate Strings(w161, "_template") -> (w171:string)
                n71 = Build Path(base path=w160, name or relative path=w171) -> (appended path=w173:path)
                n72 = call <vilib>:"Open_Create_Replace File.vi"("file path"=w173) -> ("error out"=w163:errorcluster, "refnum"=w170:refnum<file>)  [unwired: 5 in, 4 out]
                n73 = Get File Size(file=w170, error in=w163) -> (refnum out=w169:refnum<file>, size (in bytes)=w167:i64, 0:w158:errorcluster)
                n74 = Unbundle By Name(w158) -> ("status"=w164:bool)
                n75 = To Long Integer(number=w167) -> (32bit integer=w168:i32)
                n76 = Equal To 0?(x=w168) -> (x = 0?=w165:bool)
                n77 = Or(x=w165, y=w164) -> (x .or. y?=w166:bool)
                n78 = case shown="False" w166 {
                  tunnel: [w190 w195] -> w159
                  tunnel: w162 -> [w191 w194]
                  tunnel: w169 -> [w192 w195]
                  tunnel: [w187 w194] -> w157
                  tunnel: w158 -> [w189 w193]
                  tunnel: [w188 w193] -> _
                  frame False {
                    # "Read out the data file"
                    n79 = Read from Binary File(5:w191, 8:w189, 11:w192) -> (0:w188:errorcluster, 2:w187:T9, 3:w190:refnum<file>)  [unwired: 4 out]
                  }
                  frame True {
                  }
                }
                n80 = Close File(refnum=w159) -> ()  [unwired: 1 in, 2 out]
                n81 = Unbundle(w157) -> ("Master Output Bits"=w178:bool[], "Slave Output Bits"=w177:bool[], "AO Values"=w176:T1, "DO Values"=w175:T3, "Novatech settings"=w174:T4)
                n82 = local write "Master Output Bits"(w178) -> ()
                n83 = local write "Slave Output Bits"(w177) -> ()
                n84 = local write "Novatech settings"(w174) -> ()
                n85 = local write "AO Values"(w176) -> ()
                n86 = local write "DO Values"(w175) -> ()
              }
            }
          }
          event "Save": Value Change {
            n87 = event-data() -> ("NewVal"=w196:bool)  [unwired: 1 in, 4 out]
            n88 = case shown="True" w196 {
              frame False {
              }
              frame True {
                n89 = local read "Path"() -> (w200:path)
                n90 = property on="History" class="CmbBox"() -> ("Strings[]"=w216:string[])  [unwired: 2 in, 2 out]
                n91 = local write "Save"(FALSE) -> ()
                n92 = Path To String(path=w200) -> (string=w215:string)
                n93 = call "Load_SetList_HistoryUpdate_v4.vi"("New Element"=w215, "History in"=w216) -> ()  [unwired: 1 out]
                n94 = call "Load_SetList_HistoryUpdate_v4.vi"("New Element"=w215, "History in"=w216) -> ("History Out"=w197:string[])
                n95 = property on="History" class="CmbBox"("Strings[]"=w197) -> ()  [unwired: 2 in, 2 out]
                n96 = Create Folder(path (use dialog)=w200) -> (created path=w199:path)  [unwired: 1 in, 3 out]
                n97 = Strip Path(path=w200) -> (name=w201:string)  [unwired: 1 out]
                n98 = local read "Master Output Bits"() -> (w213:bool[])
                n99 = local read "Novatech settings"() -> (w209:T4)
                n100 = local read "Slave Output Bits"() -> (w212:bool[])
                n101 = local read "AO Values"() -> (w211:T1)
                n102 = local read "DO Values"() -> (w210:T3)
                n103 = Concatenate Strings(w201, "_template") -> (w203:string)
                n104 = Build Path(base path=w199, name or relative path=w203) -> (appended path=w207:path)
                n105 = call <vilib>:"Open_Create_Replace File.vi"("function (open:0)"=T6."create or replace", "file path"=w207) -> ("refnum"=w208:refnum<file>)  [unwired: 4 in, 5 out]
                n106 = Bundle("Master Output Bits"=w213, "Slave Output Bits"=w212, "AO Values"=w211, "DO Values"=w210, "Novatech settings"=w209) -> (w198:T9)  [unwired: 1 in]
                n107 = Write to Binary File(file (use dialog)=w208, data=w198, 5:TRUE ("prepend array or string size? (T)")) -> (refnum out=w205:refnum<file>)  [unwired: 1 in, 4 out]
                n108 = Close File(refnum=w205) -> ()  [unwired: 1 in, 2 out]
              }
            }
          }
        }
      }
    }
  }
  n109 = call <vilib>:"Release Semaphore_71.vi"("error in (no error)"=w9, "semaphore"=w1) -> ("error out"=w10:errorcluster, "semaphore out"=w11:T5)  [unwired: 4 out]
  n110 = call <vilib>:"Destroy Semaphore.vi"("error in (no error)"=w10, "semaphore"=w11) -> ("error out"=→"error out":errorcluster)  [unwired: 5 out]
